vi "Trial1.vi"() -> ()   [LabVIEW 2013]
doc: "This example shows how to use the driver's VI's to set up the Polaris and acquire transformations. For this example, all wired tools are activated and one wireless tool is activated."
uses:
  <vilib>/Platform/NI_3dgraph.lvlib
panel:
  in  "Location of ROM File for Tool":path=path "C:/Program Files/Northern Digital Inc/8700248.rom"
  in  "Serial Configuration":T1={"Baud Rate (9600)"=9600, "Flow Control (0:None)"=0, "Parity"=0, "Data Bits"=8, "Stop Bits"=10} {"Stop Bits" items=["1.0"=10, "2.0"=20]; "Parity" items=["None", "Odd", "Even"]; "Flow Control (0:None)" items=["None", "XON/XOFF"]; "Baud Rate (9600)" items=["9600"=9600, "14.4k"=14400, "19.2k"=19200, "38.4k"=38400, "57.6k "=57600, "115.2k"=115200]}
  out "Current Transformations":T2(array[cluster])
  in  "VISA resource name":refnum<visa-resource-name>="COM1"
  in  "Reset? (T:Yes)":bool=TRUE
  in  "3D Curve":refnum<k7>(container)
  in  "Track Outside Measurement Volume? (F:No)":bool
  in  "Plot Data? (T:Yes)":bool=TRUE
  in  "STOP":bool
  # "NOTE: This VI will only run on machines using a Windows OS (for ActiveX support).  Plotting this 3D data\nis NOT meant for performance, rather it is intended to give a more intuitive representation of the data\nreturned by the Polaris instrument.  For demonstration of faster acquisition, please take a look at the\nndipolaris Measurement Exampole VI."
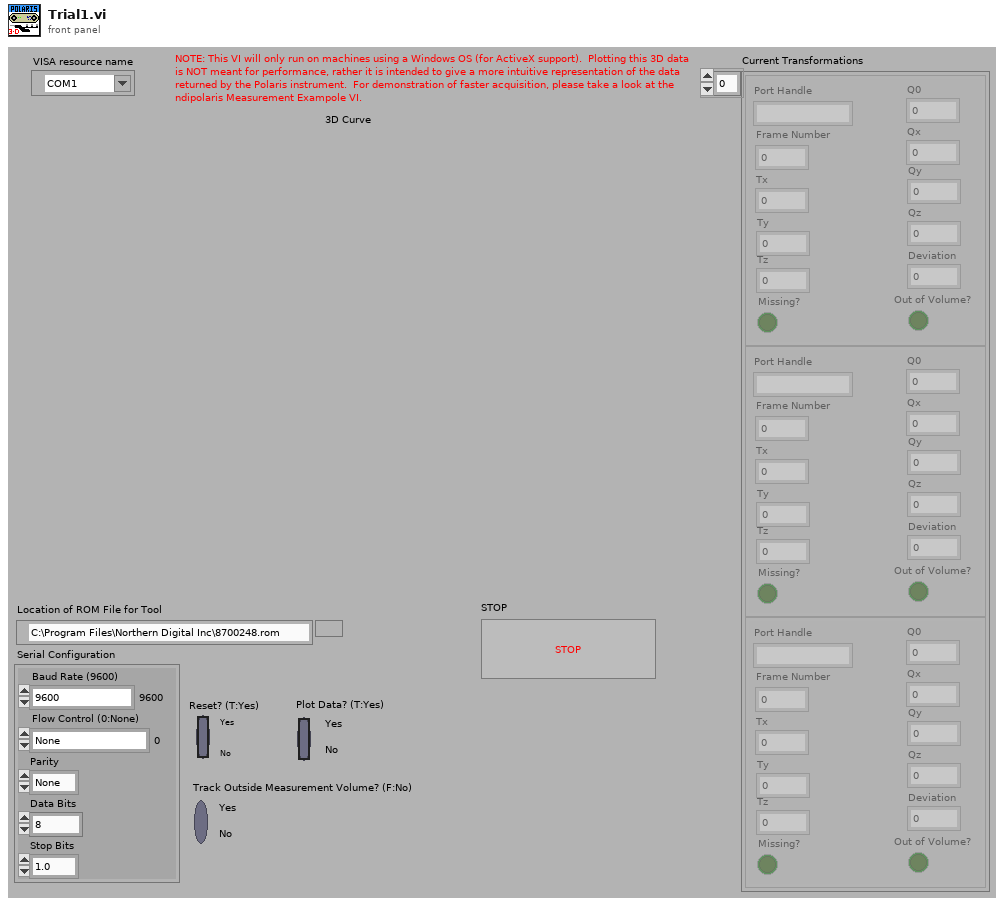
[diagram p1: front panel]
types:
  T1 = cluster{"Baud Rate (9600)":u32, "Flow Control (0:None)":u16, "Parity":u16, "Data Bits":u16, "Stop Bits":u16}
  T2 = cluster{"Port Handle":string, "Frame Number":u32, "Tx":dbl, "Ty":dbl, "Tz":dbl, "Q0":dbl, "Qx":dbl, "Qy":dbl, "Qz":dbl, "Deviation":dbl, "Missing?":bool, "Out of Volume?":bool}[]
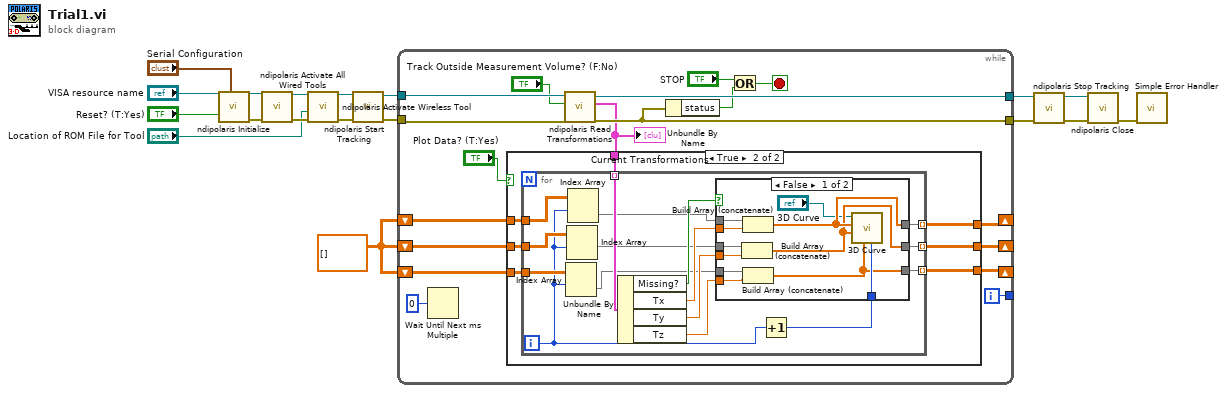
[diagram p0: block diagram]
diagram:
  w11 = dbl[][] []
  n1 = call <instrlib>:"ndipolaris Initialize.vi"("Serial Configuration"="Serial Configuration", "Reset? (T: Yes)"="Reset? (T:Yes)", "VISA resource name"="VISA resource name") -> ("error out"=w12:errorcluster, "VISA resource name out"=w13:refnum<visa-resource-name>)  [unwired: 7 in]
  n2 = call <instrlib>:"ndipolaris Activate All Wired Tools.vi"("error in (no error)"=w12, "VISA resource name"=w13) -> ("error out"=w16:errorcluster, "VISA resource out"=w17:refnum<visa-resource-name>)  [unwired: 7 in, 1 out]
  n3 = call <instrlib>:"ndipolaris Activate Wireless Tool.vi"("error in (no error)"=w16, "Location of ROM File for Tool"="Location of ROM File for Tool", "VISA resource name"=w17) -> ("error out"=w14:errorcluster, "VISA resource out"=w15:refnum<visa-resource-name>)  [unwired: 6 in, 1 out]
  n4 = call <instrlib>:"ndipolaris Start Tracking.vi"("error in (no error)"=w14, "VISA resource name"=w15) -> ("error out"=w3:errorcluster, "VISA resource out"=w4:refnum<visa-resource-name>)  [unwired: 8 in]
  n5 = while {
    tunnel: w4 -> [w36]
    tunnel: w3 -> [w35]
    tunnel: [w20] -> _
    tunnel: [w30] -> w6
    tunnel: [w29] -> w5
    shift-right: [w23] -> _
    shift-left: w11 -> [w26]
    shift-right: [w22] -> _
    shift-left: w11 -> [w25]
    shift-right: [w21] -> _
    shift-left: w11 -> [w24]
    i -> [w20]
    stop <- w33 stop-if-true
    n6 = Wait Until Next ms Multiple(millisecond multiple=u32 0) -> ()  [unwired: 1 out]
    n7 = call <instrlib>:"ndipolaris Read Transformations.vi"("error in (no error)"=w35, "Get Extended Tool Info? (F:No)"="Track Outside Measurement Volume? (F:No)", "VISA resource name"=w36) -> ("error out"=w29:errorcluster, "Transformations"=w19:T2, "VISA resource out"=w30:refnum<visa-resource-name>)  [unwired: 5 in, 1 out]
    "Current Transformations" <- w19
    n8 = case shown="True" "Plot Data? (T:Yes)" {
      tunnel: w19 -> [_ w46]
      tunnel: w26 -> [w39 w42]
      tunnel: w25 -> [w38 w41]
      tunnel: w24 -> [w37 w40]
      tunnel: [w39 w45] -> w23
      tunnel: [w38 w44] -> w22
      tunnel: [w37 w43] -> w21
      frame False {
      }
      frame True {
        n9 = for {
          tunnel: w46 -> [w62] mode=indexing
          tunnel: [w56] -> w43 mode=indexing
          tunnel: [w55] -> w44 mode=indexing
          tunnel: [w54] -> w45 mode=indexing
          tunnel: w42 -> [w53]
          tunnel: w41 -> [w51]
          tunnel: w40 -> [w52]
          i -> [w50]
          n10 = Index Array(array=w52, index (row)=w50) -> (element=w47:dbl[])  [unwired: 1 in]
          n11 = Index Array(array=w51, index (row)=w50) -> (element=w48:dbl[])  [unwired: 1 in]
          n12 = Index Array(array=w53, index (row)=w50) -> (element=w49:dbl[])  [unwired: 1 in]
          n13 = Unbundle By Name(w62) -> ("Missing?"=w61:bool, "Tx"=w60:dbl, "Ty"=w59:dbl, "Tz"=w58:dbl)
          n14 = Increment(x=w50) -> (x+1=w57:i32)
          n15 = case shown="False" w61 {
            tunnel: w60 -> [w73 _]
            tunnel: w59 -> [w72 _]
            tunnel: w58 -> [w71 _]
            tunnel: w57 -> [w70 _]
            tunnel: [w69 w76] -> w54
            tunnel: [w68 w75] -> w55
            tunnel: [w67 w74] -> w56
            tunnel: w49 -> [w66 w76]
            tunnel: w48 -> [w65 w75]
            tunnel: w47 -> [w64 w74]
            frame False {
              n16 = Build Array (concatenate)(w65, w72) -> (w68:dbl[])
              n17 = Build Array (concatenate)(w66, w73) -> (w69:dbl[])
              n18 = Build Array (concatenate)(w64, w71) -> (w67:dbl[])
              n19 = call <vilib>:"3D Curve.vi"("plot number (1)"=w70, "z vector"=w67, "y vector"=w68, "x vector"=w69, "3D graph"="3D Curve") -> ()  [unwired: 5 in, 2 out]
            }
            frame True {
            }
          }
        }
      }
    }
    n20 = Unbundle By Name(w29) -> ("status"=w28:bool)
    n21 = Or(x="STOP", y=w28) -> (x .or. y?=w33:bool)
  }
  n22 = call <instrlib>:"ndipolaris Stop Tracking.vi"("error in (no error)"=w5, "VISA resource name"=w6) -> ("error out"=w8:errorcluster, "VISA resource out"=w9:refnum<visa-resource-name>)  [unwired: 8 in]
  n23 = call <instrlib>:"ndipolaris Close.vi"("error in (no error)"=w8, "VISA resource name"=w9) -> ("error out"=w7:errorcluster)  [unwired: 9 in]
  n24 = call <vilib>:"Simple Error Handler.vi"("error in (no error)"=w7) -> ()  [unwired: 4 in, 5 out]
